vi "extract-value.vi"(2 "Variable":string, 3 "Chaine contenant valeur":string) -> (0 "Valeur":dbl, 1 "Valeur en string":string)   [LabVIEW 2018]
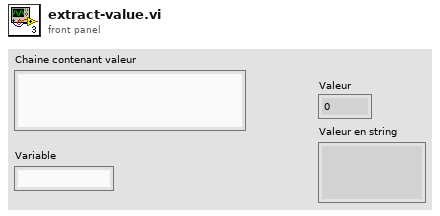
[diagram p1: front panel]
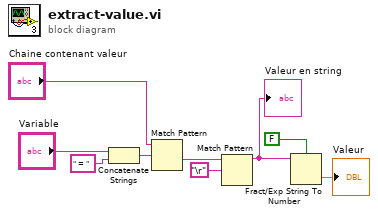
[diagram p0: block diagram]
diagram:
  n1 = Concatenate Strings("Variable", " = " ("regular expression")) -> (w5:string)
  n2 = Match Pattern(string="Chaine contenant valeur", regular expression=w5) -> (after substring=w9:string)  [unwired: 1 in, 3 out]
  n3 = Match Pattern(string=w9, regular expression="\r") -> (before substring=w2:string)  [unwired: 1 in, 3 out]
  "Valeur en string" <- w2
  n4 = Fract/Exp String To Number(use system decimal point (T)=FALSE ("utiliser le séparateur décimal du système (V)"), string=w2) -> (number=→"Valeur":dbl)  [unwired: 2 in, 1 out]
